vi "T7Inclinometer.vi"(11 "T7InclinometerSettings":T1={"SerialPort"="RS232\\Port1", "TimestampRegister"="TimestampRegister", "TxFIFO"="T7InclinometerTxFIFO", "RxFIFO"="T7InclinometerRxFIFO"}) -> ()   [LabVIEW 2016, in "FPGAT7Inclinometer.lvlib"]
uses:
  FPGAT7Inclinometer.lvlib
  DataTypes/T7InclinometerSettings.ctl
  <vilib>/rvi/Emulation/niFpgaGetClockAttributes.vi
  <vilib>/rvi/Emulation/niFpgaSctlEmulationGetInTimedLoop.vi
  <vilib>/rvi/Emulation/niFpgaEmulationReportErrorSimple.vi
  <vilib>/rvi/DataTransferAndStorage/Container/Common/niFpgaContainerExecOnDevCompGetState.vi
  <vilib>/rvi/Emulation/niFpgaEmulationIsFPGAContextNoSignature.vi
  <vilib>/rvi/errors/niFpgaSetErrorForExecOnDevCompSimple.vi
  <vilib>/rvi/eio/common/nirviEmuReportErrorAndStop.vi
  <vilib>/rvi/DataTransferAndStorage/Container/Common/niFpgaContainerGetUniqueNameForEmu.vi
  <vilib>/rvi/FIFO/Fifo_Resource/nirvififoEmulationSetSize.vi
  <vilib>/rvi/FIFO/Fifo_Resource/nirviFifoEmulationQueueMgr.vi
  <instcachedir>/0/nirviFifoEmulationQueueMgr_E5CAEC123FF24DC58D834DCA3CDAA9B5.lvgen/nirviFifoEmulationQueueMgr_E5CAEC123FF24DC58D834DCA3CDAA9B5_009.vi
  <vilib>/rvi/FIFO/Fifo_Resource/nirvififoEmulationDetermineInputValidOut.vi
  <vilib>/rvi/FIFO/Fifo_Resource/nirvififoEmulationCreateLock.vi
  <vilib>/rvi/Emulation/niFpgaProcessEmulError.vi
  <vilib>/rvi/FIFO/Fifo_Resource/nirvififoEmulationObtainLock.vi
  <vilib>/rvi/FIFO/Fifo_Resource/nirvififoEmulationReleaseLock.vi
  <vilib>/rvi/occurrence/nirviWaitOnOccurrenceBase.vi
  <vilib>/rvi/errors/nirviReportUnexpectedCaseInternalError.vi
  <vilib>/rvi/errors/nirviReportUnexpectedCaseInternalError (U32).vi
  <vilib>/Utility/error.llb/Clear Errors.vi
  <vilib>/rvi/interface/RandomDataEmulation/niFpgaRandomDataHandleErrors.vi
  <vilib>/rvi/eio/common/nirviEmuTemplateMethod_errors.vi
  <vilib>/rvi/Memory/Memory_Emulation/niFpgaMemoryEmulationCacheClearOnFirstRun.vi
  <vilib>/rvi/Memory/Memory_Emulation/nirvimemoryEmulationManagerCache_MakeExclusive.vi
  <vilib>/rvi/Memory/Memory_Emulation/niFpgaMemoryEmulationValidateCache.vi
  <vilib>/rvi/Memory/Memory_Emulation/nirvimemoryEmulationManagerCache_InsertValue.vi
  <vilib>/rvi/Memory/Memory_Emulation/nirvimemoryEmulationManagerCache_ReleaseExclusive.vi
  <vilib>/rvi/Memory/Memory_Emulation/nirvimemoryEmulationManagerCache_GetValue.vi
  <vilib>/rvi/Memory/Memory_Emulation/nirvimemoryEmulationManagerCache_SetValue.vi
  <vilib>/rvi/Emulation/niFpgaCriticalErrorInLSC.vi
  <vilib>/rvi/DataTransferAndStorage/Container/XNode/niFpgaContainer.xnode
  <vilib>/rvi/FIFO/Fifo_Resource/niFpgaFifoEmulationRefIn.vi
  <vilib>/eio/EIOMethodNode/EIOMethodNode.xnode
  <vilib>/rvi/DataTransferAndStorage/Register/Emulation/niFpgaRegisterEmulationRefIn.vi
  Common_FPGA_FIFO/FPGAFIFO.lvlib
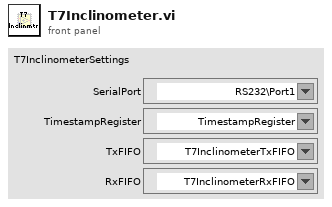
[diagram p1: front panel]
types:
  T1 = typedef "FPGAT7Inclinometer.lvlib/T7InclinometerSettings.ctl" = cluster{"SerialPort":refnum<k21>, "TimestampRegister":refnum<k21>, "TxFIFO":refnum<k21>, "RxFIFO":refnum<k21>}
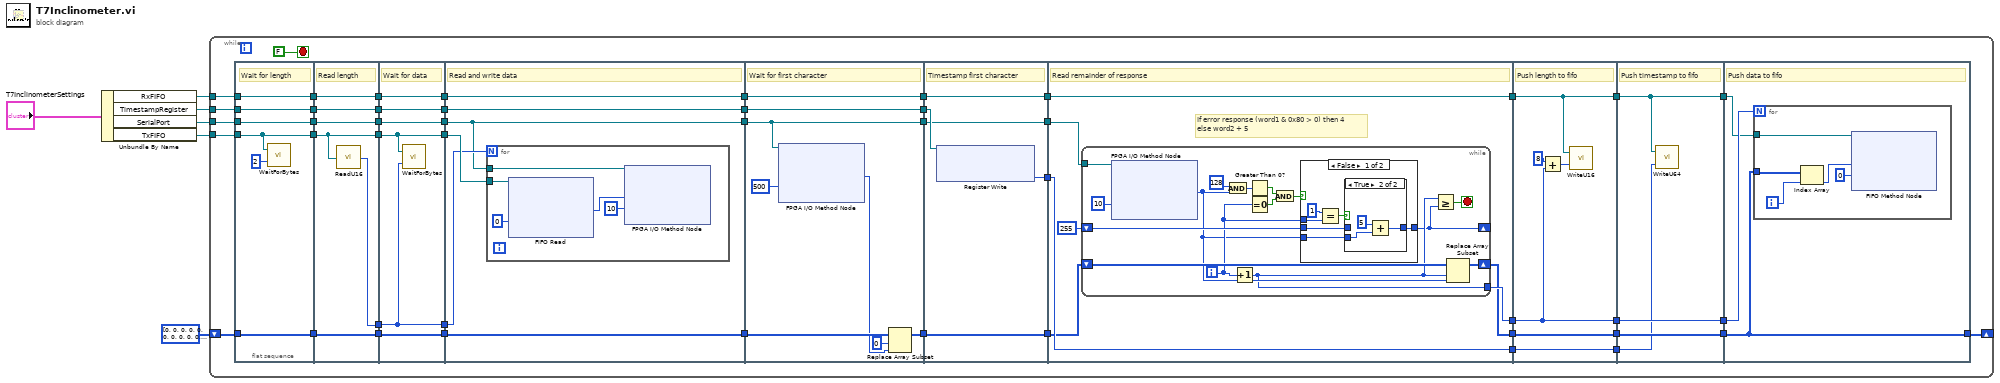
[diagram p0: block diagram]
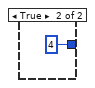
[diagram p3: hidden frame]
diagram:
  n1 = Unbundle By Name("T7InclinometerSettings") -> ("RxFIFO"=w3:refnum<k21>, "TimestampRegister"=w5:refnum<k21>, "SerialPort"=w6:refnum<k21>, "TxFIFO"=w2:refnum<k21>)
  n2 = while {
    tunnel: w6 -> [w53]
    tunnel: w5 -> [w52]
    shift-right: [w45] -> _
    shift-left: u8[] [0, 0, 0, 0, 0, 0, 0, 0, 0, 0, 0, 0, 0, 0, 0, 0, 0, 0, 0, 0, 0, 0, 0, 0, 0, 0, 0, 0, 0, 0, 0, 0, 0, 0, 0, 0, 0, 0, 0, 0, 0, 0, 0, 0, 0, 0, 0, 0, 0, 0, 0, 0, 0, 0, 0, 0, 0, 0, 0, 0, 0, 0, 0, 0, 0, 0, 0, 0, 0, 0, 0, 0, 0, 0, 0, 0, 0, 0, 0, 0, 0, 0, 0, 0, 0, 0, 0, 0, 0, 0, 0, 0, 0, 0, 0, 0, 0, 0, 0, 0, 0, 0, 0, 0, 0, 0, 0, 0, 0, 0, 0, 0, 0, 0, 0, 0, 0, 0, 0, 0, 0, 0, 0, 0, 0, 0, 0, 0, 0, 0, 0, 0, 0, 0, 0, 0, 0, 0, 0, 0, 0, 0, 0, 0, 0, 0, 0, 0, 0, 0, 0, 0, 0, 0, 0, 0, 0, 0, 0, 0, 0, 0, 0, 0, 0, 0, 0, 0, 0, 0, 0, 0, 0, 0, 0, 0, 0, 0, 0, 0, 0, 0, 0, 0, 0, 0, 0, 0, 0, 0, 0, 0, 0, 0, 0, 0, 0, 0, 0, 0, 0, 0, 0, 0, 0, 0, 0, 0, 0, 0, 0, 0, 0, 0, 0, 0, 0, 0, 0, 0, 0, 0, 0, 0, 0, 0, 0, 0, 0, 0, 0, 0, 0, 0, 0, 0, 0, 0, 0, 0, 0, 0, 0, 0, 0, 0, 0, 0, 0, 0, 0, 0, 0, 0, 0, 0] -> [w49]
    tunnel: w3 -> [w47]
    tunnel: w2 -> [w37]
    stop <- FALSE stop-if-true
    n3 = flat-sequence {
      tunnel: w37 -> [w54]
      tunnel: w47 -> [w56]
      tunnel: w49 -> [w57]
      tunnel: w52 -> [w58]
      tunnel: w53 -> [w59]
      tunnel: [w59] -> w36
      tunnel: [w58] -> w35
      tunnel: [w57] -> w34
      tunnel: [w56] -> w33
      tunnel: [w54] -> w32
      tunnel: w36 -> [w65]
      tunnel: [w65] -> w31
      tunnel: w35 -> [w64]
      tunnel: [w64] -> w29
      tunnel: w34 -> [w63]
      tunnel: [w63] -> w27
      tunnel: w33 -> [w62]
      tunnel: [w62] -> w25
      tunnel: w32 -> [w61]
      tunnel: [w61] -> w23
      tunnel: [w60] -> w21
      tunnel: w31 -> [w71]
      tunnel: [w71] -> w30
      tunnel: w29 -> [w70]
      tunnel: [w70] -> w28
      tunnel: w27 -> [w69]
      tunnel: [w69] -> w26
      tunnel: w25 -> [w68]
      tunnel: [w68] -> w24
      tunnel: w23 -> [w66]
      tunnel: [w66] -> w22
      tunnel: w21 -> [w67]
      tunnel: [w67] -> w20
      tunnel: [w73] -> w19
      tunnel: [w77] -> w17
      tunnel: [w76] -> w14
      tunnel: w30 -> [w73]
      tunnel: w28 -> [w77]
      tunnel: w26 -> [w72]
      tunnel: w24 -> [w76]
      tunnel: w22 -> [w75]
      tunnel: w20 -> [w74]
      tunnel: [w72] -> w12
      tunnel: w19 -> [w83]
      tunnel: [w83] -> w18
      tunnel: w17 -> [w90]
      tunnel: [w90] -> w16
      tunnel: [w85] -> w15
      tunnel: w14 -> [w89]
      tunnel: [w89] -> w13
      tunnel: w12 -> [w86]
      tunnel: w18 -> [w93]
      tunnel: w16 -> [w95]
      tunnel: [w94] -> w51
      tunnel: [w93] -> w50
      tunnel: w15 -> [w92]
      tunnel: [w92] -> w48
      tunnel: w13 -> [w91]
      tunnel: [w91] -> w46
      tunnel: w51 -> [w99]
      tunnel: w50 -> [w102]
      tunnel: w48 -> [w98]
      tunnel: [w101] -> w43
      tunnel: w46 -> [w100]
      tunnel: [w100] -> w42
      tunnel: [w99] -> w11
      tunnel: [w97] -> w9
      tunnel: w43 -> [w134]
      tunnel: [w134] -> w41
      tunnel: w42 -> [w130]
      tunnel: [w130] -> w39
      tunnel: w11 -> [w131]
      tunnel: [w132] -> w10
      tunnel: w9 -> [w132]
      tunnel: [w131] -> w7
      tunnel: w41 -> [w138]
      tunnel: [w138] -> w40
      tunnel: w39 -> [w136]
      tunnel: [w136] -> w38
      tunnel: w10 -> [w137]
      tunnel: [w137] -> w8
      tunnel: w7 -> [w135]
      tunnel: w40 -> [w141]
      tunnel: w38 -> [w140]
      tunnel: [w139] -> w45
      tunnel: w8 -> [w139]
      frame #0 {
        # "Wait for length"
        n4 = call "WaitForBytes.vi"("Bytes"=u16 2, "FIFO"=w54) -> ()  [unwired: 1 in]
      }
      frame #1 {
        # "Read length"
        n5 = call "ReadU16.vi"("FIFO"=w61) -> ("U16"=w60:u16)
      }
      frame #2 {
        # "Wait for data"
        n6 = call "WaitForBytes.vi"("Bytes"=w67, "FIFO"=w66) -> ()  [unwired: 1 in]
      }
      frame #3 {
        # "Read and write data"
        n7 = for {
          N: w74 -> [_]
          tunnel: w75 -> [w82]
          tunnel: w73 -> [w80]
          n8 = xnode "FIFO Read"("Timeout"=0, "FIFO In"=w82) -> ("Element"=w79:u8)  [unwired: 2 out]
          n9 = xnode "FPGA I/O Method Node"("FPGA I/O In"=w80, "Data"=w79, "Timeout (ms)"=10) -> ()  [unwired: 2 out]
        }
      }
      frame #4 {
        # "Wait for first character"
        n10 = xnode "FPGA I/O Method Node"("FPGA I/O In"=w83, "Timeout (ms)"=500) -> ("Data"=w84:u8)  [unwired: 2 out]
        n11 = Replace Array Subset(array=w86, new element=w84, index=0) -> (w85:u8[])
      }
      frame #5 {
        # "Timestamp first character"
        n12 = xnode "Register Write"("Register In"=w95) -> ("Data"=w94:u64)  [unwired: 1 out]
      }
      frame #6 {
        # "If error response (word1 & 0x80 > 0) then 4\nelse word2 + 5"
        # "Read remainder of response"
        n13 = while {
          tunnel: w102 -> [w117]
          shift-right: [w115] -> w97
          shift-left: w98 -> [w116]
          tunnel: [w105] -> w101
          shift-right: [w104] -> _
          shift-left: u8 255 -> [w108]
          i -> [w107]
          stop <- w103 stop-if-true
          n14 = xnode "FPGA I/O Method Node"("FPGA I/O In"=w117, "Timeout (ms)"=10) -> ("Data"=w106:u8)  [unwired: 2 out]
          n15 = And(x=u8 128, y=w106) -> (x .and. y?=w112:u8)
          n16 = Increment(x=w107) -> (x+1=w105:i32)
          n17 = Greater Than 0?(x=w112) -> (x > 0?=w111:bool)
          n18 = Equal To 0?(x=w107) -> (x = 0?=w110:bool)
          n19 = And(x=w111, y=w110) -> (x .and. y?=w109:bool)
          n20 = case shown="False" w109 {
            tunnel: w108 -> [w119 _]
            tunnel: w107 -> [w123 _]
            tunnel: [w120 u8 4] -> w104
            tunnel: w106 -> [w118 _]
            frame False {
              n21 = Equal?(x=1, y=w123) -> (x = y?=w121:bool)
              n22 = case shown="True" w121 {
                tunnel: [w124 w125] -> w120
                tunnel: w119 -> [w124 _]
                tunnel: w118 -> [_ w127]
                frame False {
                }
                frame True {
                  n23 = Add(x=u8 5, y=w127) -> (x+y=w125:u8)
                }
              }
            }
            frame True {
            }
          }
          n24 = Greater Or Equal?(x=w105, y=w104) -> (x >= y?=w103:bool)
          n25 = Replace Array Subset(array=w116, new element=w106, index=w105) -> (w115:u8[])
        }
      }
      frame #7 {
        # "Push length to fifo"
        n26 = Add(x=8, y=w134) -> (x+y=w129:i32)
        n27 = call "WriteU16.vi"("U16"=w129, "FIFO"=w130) -> ()  [unwired: 1 in]
      }
      frame #8 {
        # "Push timestamp to fifo"
        n28 = call "WriteU64.vi"("U64"=w135, "FIFO"=w136) -> ()  [unwired: 1 in]
      }
      frame #9 {
        # "Push data to fifo"
        n29 = for {
          N: w141 -> [_]
          tunnel: w139 -> [w146]
          tunnel: w140 -> [w145]
          i -> [w143]
          n30 = Index Array(array=w146, index=w143) -> (element=w144:u8)
          n31 = xnode ("FIFO Method Node")("Element"=w144, "Timeout"=0, "FIFO In"=w145) -> ()  [unwired: 2 out]
        }
      }
    }
  }
